vi "addI32Element.vi"(7 "Name":string, 8 "error in (no error)":errorcluster, 9 "Value":i32, 10 "Replace? (false)":bool, 11 "tBSONDocument in":refnum<class "tBSONDocument.lvclass">) -> (0 "error out":errorcluster, 3 "tBSONDocument out":refnum<class "tBSONDocument.lvclass">)   [LabVIEW 2013, in "BSON.lvlib" / "tBSONDocument.lvclass"]
doc: "Adds an I32 to a BSON document."
uses:
  tBSONDocument.lvclass
  BSONElements/tBSON_I32/tBSON_I32.lvclass
  tBSONElement/tBSONElement.lvclass
  tBSONElement/setName.vi
  BSONElements/tBSON_I32/setValue.vi
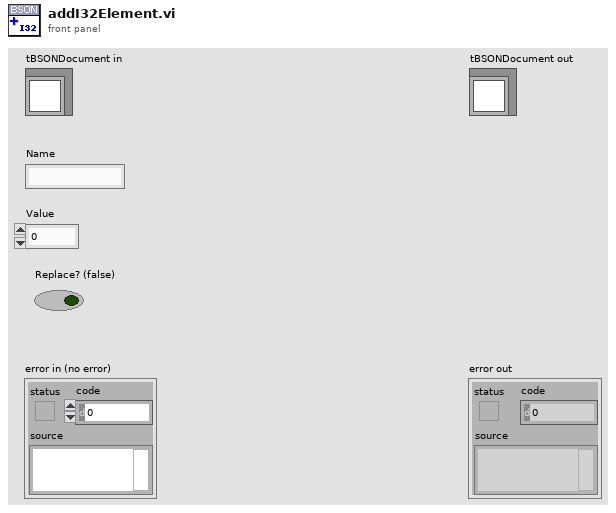
[diagram p1: front panel]
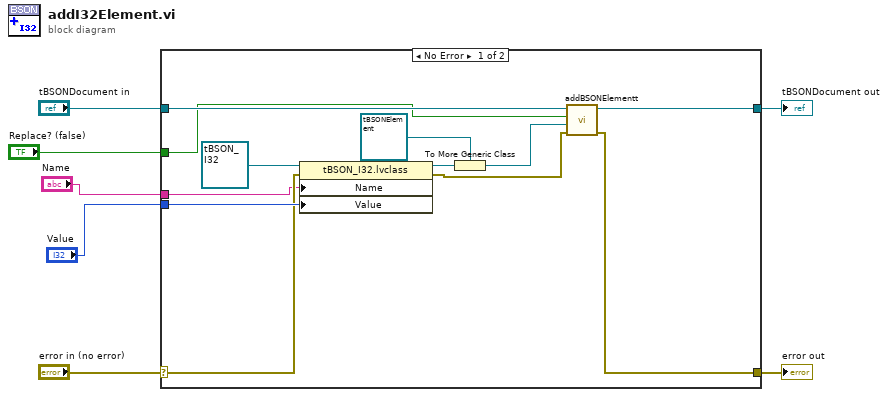
[diagram p0: block diagram]
diagram:
  n1 = case shown="No Error" "error in (no error)" {
    selector: "error in (no error)" -> [w17 w21]
    tunnel: [w11 w21] -> w6
    tunnel: [w13 w20] -> w4
    tunnel: "tBSONDocument in" -> [w14 w20]
    tunnel: "Value" -> [w18 _]
    tunnel: "Name" -> [w9 _]
    tunnel: "Replace? (false)" -> [w8 _]
    frame No Error {
      n2 = property class="tBSON_I32.lvclass"(reference=refnum<class "tBSON_I32.lvclass"> refnum ("BSON.lvlib:tBSON_I32.lvclass"), error in=w17, "Name"=w9, "Value"=w18) -> (reference out=w16:refnum<class "tBSON_I32.lvclass">, error out=w12:errorcluster)
      n3 = To More Generic Class(target class=refnum<class "tBSONElement.lvclass"> refnum ("BSON.lvlib:tBSONElement.lvclass"), reference=w16) -> (generic class reference=w10:refnum<class "tBSONElement.lvclass">)
      n4 = call "addBSONElementt.vi"("error in (no error)"=w12, "Element"=w10, "Replace? (false)"=w8, "tBSONDocument in"=w14) -> ("error out"=w11:errorcluster, "tBSONDocument out"=w13:refnum<class "tBSONDocument.lvclass">)  [unwired: 6 in]
    }
    frame Error {
    }
  }
  "error out" <- w6
  "tBSONDocument out" <- w4
